vi "Get Group Channels.vi"(8 "error in":errorcluster, 10 "Group selection":string, 11 "TDMS in":refnum<class "TDMS.lvclass">) -> (0 "error out":errorcluster, 1 "Channels":string[](array[string]), 2 "Group Details":T1, 3 "TDMS out":refnum<class "TDMS.lvclass">)   [LabVIEW 2019, in "TDMS.lvlib" / "TDMS.lvclass"]
uses:
  TDMS.lvclass
  Custom Controls/Group Properties.ctl
  Custom Controls/Channel Properties.ctl
  TDMS.lvclass/TDMS.ctl
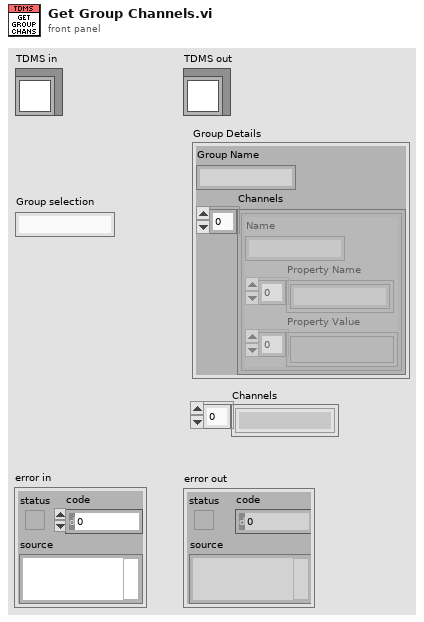
[diagram p1: front panel]
types:
  T1 = typedef "TDMS.lvlib/TDMS.lvclass/Group Properties.ctl" = cluster{"Group Name":string, "Channels":T2[]}
  T2 = typedef "TDMS.lvlib/TDMS.lvclass/Channel Properties.ctl" = cluster{"Name":string, "Property Name":string[], "Property Value":variant[]}
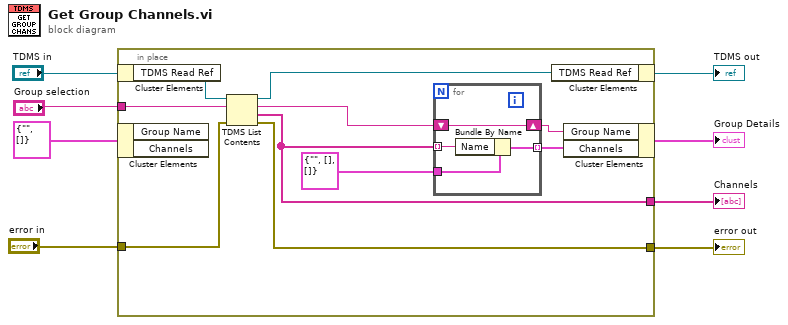
[diagram p0: block diagram]
diagram:
  n1 = in-place {
    in-place-border: "error in" -> [w16]
    in-place-border: [w15] -> w5
    in-place-border: "Group selection" -> [w14]
    in-place-border: [w9] -> w1
    n2 = in-place-cluster #1("TDMS in") -> ("TDMS Read Ref"=w18:refnum<k34>)
    n3 = in-place-cluster #2(T1 {"Group Name"="", "Channels"=[]} ("Group Details")) -> ()  [unwired: 2 out]
    n4 = TDMS List Contents(4:w16, 6:w14, 7:w18) -> (0:w15:errorcluster, 1:w9:string[], 2:w11:string, 3:w17:refnum<k34>)
    n5 = for {
      tunnel: w9 -> [w21] mode=indexing
      tunnel: T2 {"Name"="", "Property Name"=[], "Property Value"=[]} ("Channel Details") -> [w22]
      tunnel: [w20] -> w12 mode=indexing
      shift-right: [w19] -> w10
      shift-left: w11 -> [w19]
      n6 = Bundle By Name(cluster=w22, "Name"=w21) -> (w20:T2)
    }
    n7 = in-place-cluster #1("TDMS Read Ref"=w17) -> (→"TDMS out":refnum<class "TDMS.lvclass">)
    n8 = in-place-cluster #2("Group Name"=w10, "Channels"=w12) -> (→"Group Details":T1)
  }
  "error out" <- w5
  "Channels" <- w1
